vi "MAIN.vi"() -> ()   [LabVIEW 2019]
panel:
  out "x+y":dbl[](array[numeric])
  out "Waveform Graph":dbl[](graph)
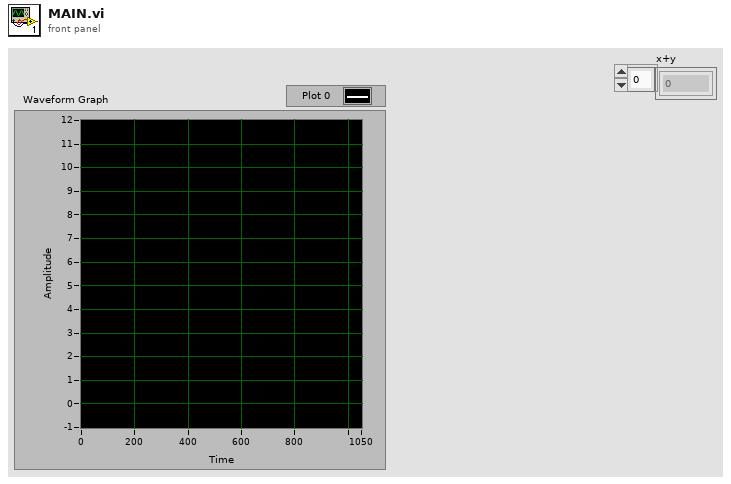
[diagram p1: front panel]
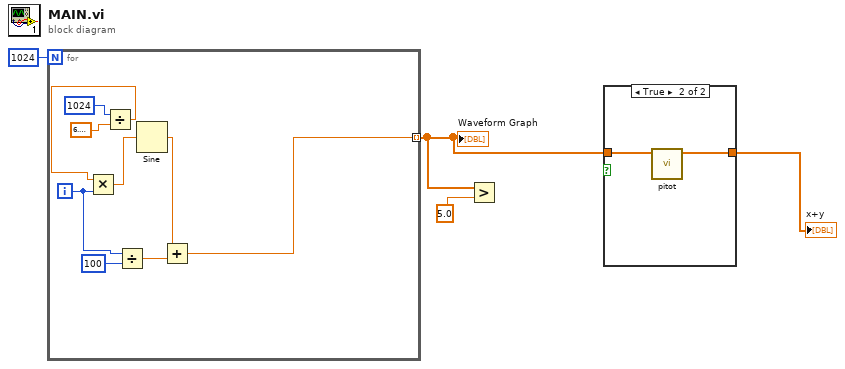
[diagram p0: block diagram]
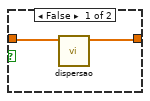
[diagram p2: hidden frame]
diagram:
  n1 = for {
    N: 1024 -> [_]
    tunnel: [w6] -> w2 mode=indexing
    i -> [w5]
    n2 = Divide(x=1024, y=6.283185307179586) -> (x/y=w11:dbl)
    n3 = Multiply(x=w11, y=w5) -> (x*y=w12:dbl)
    n4 = Divide(x=w5, y=100) -> (x/y=w8:dbl)
    n5 = Sine(x=w12) -> (sin(x)=w7:dbl)
    n6 = Add(x=w7, y=w8) -> (x+y=w6:dbl)
  }
  "Waveform Graph" <- w2
  n7 = Greater?(x=w2, y=5.0) -> ()  [unwired: 1 out]
  n8 = case shown="True" {
    selector: _ -> [_ _]
    tunnel: w2 -> [w15 w17]
    tunnel: [w14 w16] -> w1
    frame False {
      n9 = call "dispersao.vi"("Array in"=w15) -> ("Array out"=w14:dbl[])  [unwired: 10 in]
    }
    frame True {
      n10 = call "pitot.vi"("Array in"=w17) -> ("Array out"=w16:dbl[])  [unwired: 10 in]
    }
  }
  "x+y" <- w1
